vi "Format RunningInstancesItemType_LVXML_Loop.vi"(8 "error in (no error)":errorcluster, 10 "Siblings in":T2(array[cluster]), 11 "AWS_EC2 in":refnum<class "AWS_EC2.lvclass">) -> (0 "error out":errorcluster, 2 "Array":T3[](array[typedef]), 3 "AWS_EC2 out":refnum<class "AWS_EC2.lvclass">)   [LabVIEW 2014, in "AWS_EC2.lvlib" / "AWS_EC2.lvclass"]
uses:
  AWS_EC2.lvclass
  EC2 Datatypes/RunningInstancesItemsType.ctl
  EC2 Datatypes/InstanceStateType.ctl
  EC2 Datatypes/ProductCodeSetItemType.ctl
  EC2 Datatypes/PlacementResponseType.ctl
  EC2 Datatypes/GroupItemTypeSet.ctl
  EC2 Datatypes/GroupItemType.ctl
  EC2 Datatypes/StateReasonType.ctl
  EC2 Datatypes/InstanceBlockDeviceMappingResponseItemType.ctl
  EC2 Datatypes/EbsInstanceBlockDeviceMappingResponseType.ctl
  EC2 Datatypes/ResourceTagSetItemType.ctl
  EC2 Datatypes/InstanceNetworkInterfaceSetItemType.ctl
  EC2 Datatypes/InstanceNetworkInterfaceAttachmentType.ctl
  EC2 Datatypes/InstanceNetworkInterfaceAssociationType.ctl
  EC2 Datatypes/InstancePrivateIpAddressesSetItemType.ctl
  EC2 Datatypes/IamInstanceProfileResponseType.ctl
  lv-xml-parser/r0/trunk/VI Source/EventType.ctl
  AWS_EC2.lvlib
  AWS Core Lib/VI Source/AWS_Core.lvlib
  lv-xml-parser/r0/trunk/VI Source/LV XML Parser.lvlib
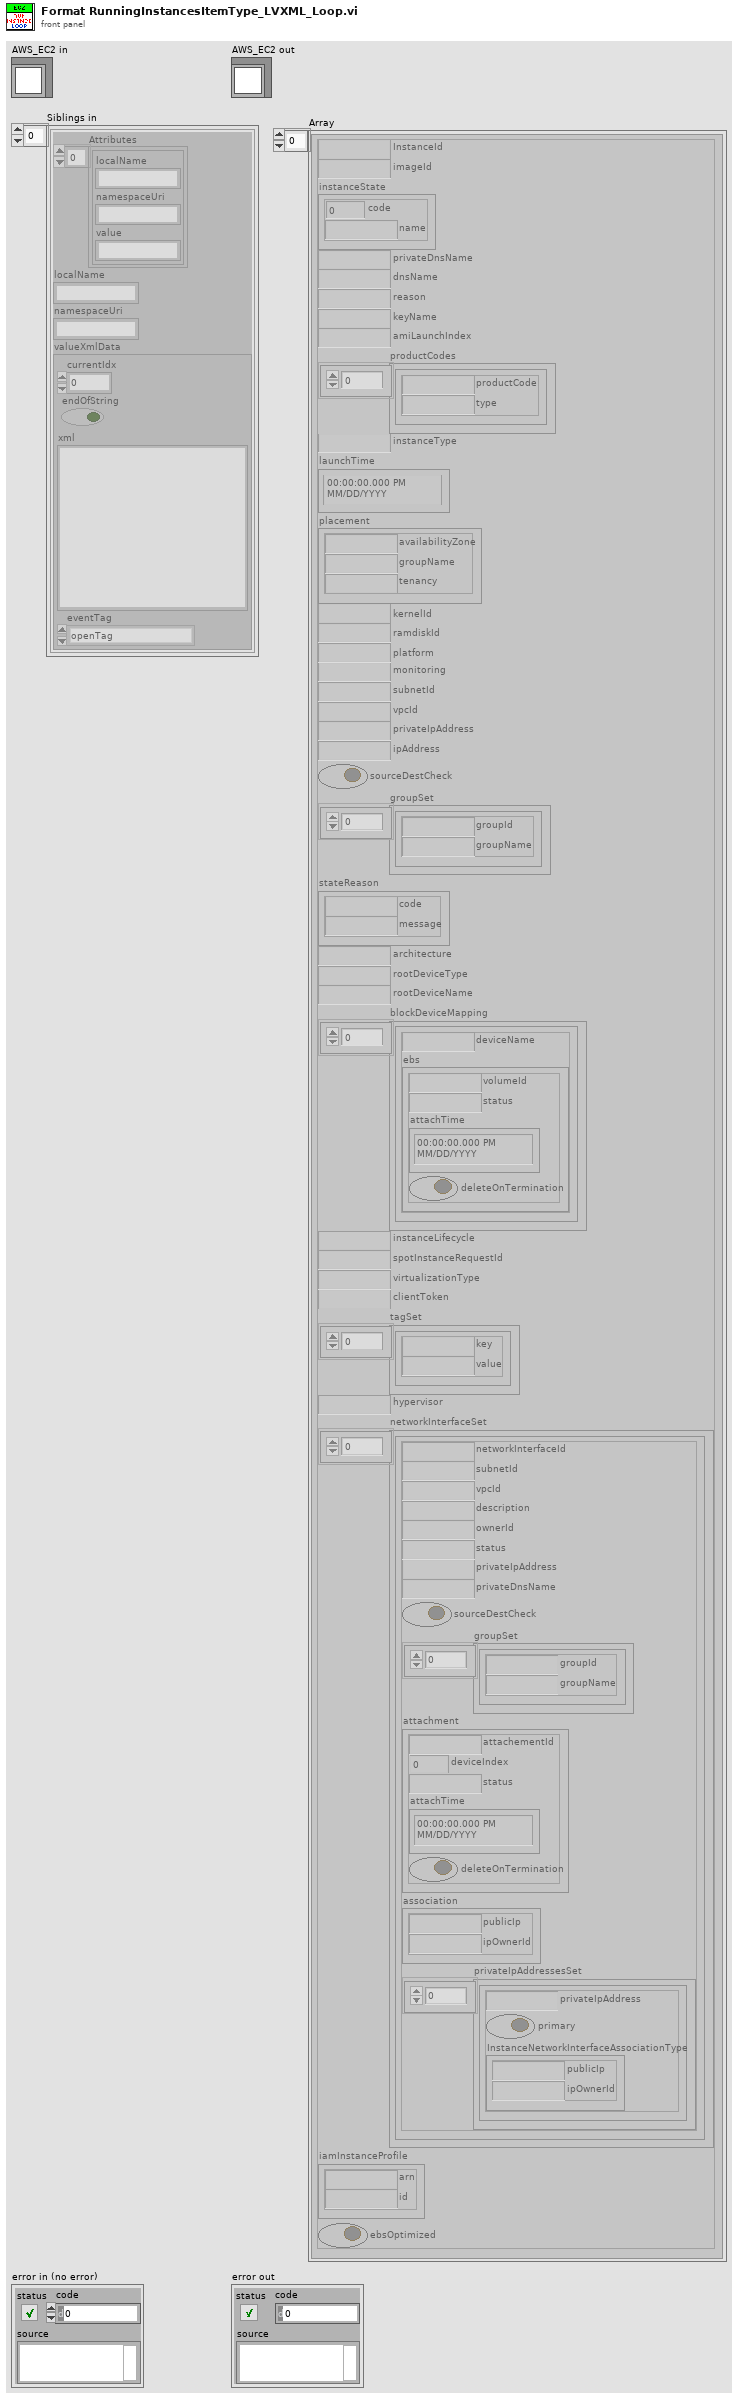
[diagram p1: front panel]
types:
  T1 = typedef "LV XML Parser.lvlib/EventType.ctl" = enum16{"openTag", "endOpenTag", "closeTag", "comment", "endComment", "endOfFile", "attribute", "startXml", "selfClosingTag"}
  T2 = cluster{"Attributes":cluster{"localName":string, "namespaceUri":string, "value":string}[], "localName":string, "namespaceUri":string, "valueXmlData":cluster{"currentIdx":i32, "endOfString":bool, "xml":string, "eventTag":T1}}[]
  T3 = typedef "AWS_EC2.lvlib/RunningInstancesItemsType.ctl" = cluster{"InstanceId":string, "imageId":string, "instanceState":T4, "privateDnsName":string, "dnsName":string, "reason":string, "keyName":string, "amiLaunchIndex":string, "productCodes":T5[], "instanceType":string, "launchTime":timestamp, "placement":T6, "kernelId":string, "ramdiskId":string, "platform":string, "monitoring":string, "subnetId":string, "vpcId":string, "privateIpAddress":string, "ipAddress":string, "sourceDestCheck":bool, "groupSet":T7, "stateReason":T9, "architecture":string, "rootDeviceType":string, "rootDeviceName":string, "blockDeviceMapping":T10[], "instanceLifecycle":string, "spotInstanceRequestId":string, "virtualizationType":string, "clientToken":string, "tagSet":T12[], "hypervisor":string, "networkInterfaceSet":T13[], "iamInstanceProfile":T17, "ebsOptimized":bool}
  T4 = typedef "AWS_EC2.lvlib/InstanceStateType.ctl" = cluster{"code":i16, "name":string}
  T5 = typedef "AWS_EC2.lvlib/ProductCodeSetItemType.ctl" = cluster{"productCode":string, "type":string}
  T6 = typedef "AWS_EC2.lvlib/PlacementResponseType.ctl" = cluster{"availabilityZone":string, "groupName":string, "tenancy":string}
  T7 = typedef "AWS_EC2.lvlib/GroupItemTypeSet.ctl" = T8[]
  T8 = typedef "AWS_EC2.lvlib/GroupItemType.ctl" = cluster{"groupId":string, "groupName":string}
  T9 = typedef "AWS_EC2.lvlib/StateReasonType.ctl" = cluster{"code":string, "message":string}
  T10 = typedef "AWS_EC2.lvlib/InstanceBlockDeviceMappingResponseItemType.ctl" = cluster{"deviceName":string, "ebs":T11}
  T11 = typedef "AWS_EC2.lvlib/EbsInstanceBlockDeviceMappingResponseType.ctl" = cluster{"volumeId":string, "status":string, "attachTime":timestamp, "deleteOnTermination":bool}
  T12 = typedef "AWS_EC2.lvlib/ResourceTagSetItemType.ctl" = cluster{"key":string, "value":string}
  T13 = typedef "AWS_EC2.lvlib/InstanceNetworkInterfaceSetItemType.ctl" = cluster{"networkInterfaceId":string, "subnetId":string, "vpcId":string, "description":string, "ownerId":string, "status":string, "privateIpAddress":string, "privateDnsName":string, "sourceDestCheck":bool, "groupSet":T7, "attachment":T14, "association":T15, "privateIpAddressesSet":T16[]}
  T14 = typedef "AWS_EC2.lvlib/InstanceNetworkInterfaceAttachmentType.ctl" = cluster{"attachementId":string, "deviceIndex":i32, "status":string, "attachTime":timestamp, "deleteOnTermination":bool}
  T15 = typedef "AWS_EC2.lvlib/InstanceNetworkInterfaceAssociationType.ctl" = cluster{"publicIp":string, "ipOwnerId":string}
  T16 = typedef "AWS_EC2.lvlib/InstancePrivateIpAddressesSetItemType.ctl" = cluster{"privateIpAddress":string, "primary":bool, "InstanceNetworkInterfaceAssociationType":T15}
  T17 = typedef "AWS_EC2.lvlib/IamInstanceProfileResponseType.ctl" = cluster{"arn":string, "id":string}
  T18 = cluster{"Attributes":cluster{"localName":string, "namespaceUri":string, "value":string}[], "localName":string, "namespaceUri":string, "valueXmlData":cluster{"currentIdx":i32, "endOfString":bool, "xml":string, "eventTag":T1}}
  T19 = cluster{"currentIdx":i32, "endOfString":bool, "xml":string, "eventTag":T1}
  T20 = cluster{"namespaceUri":string, "localName":string}
  T21 = cluster{"Attributes":cluster{"localName":string, "namespaceUri":string, "value":string}[], "localName":string, "namespaceUri":string, "valueXmlData":cluster{"currentIdx":i64, "endOfString":bool, "xml":string, "eventTag":T1}}[]
  T22 = cluster{"currentIdx":i64, "endOfString":bool, "xml":string, "eventTag":T1}
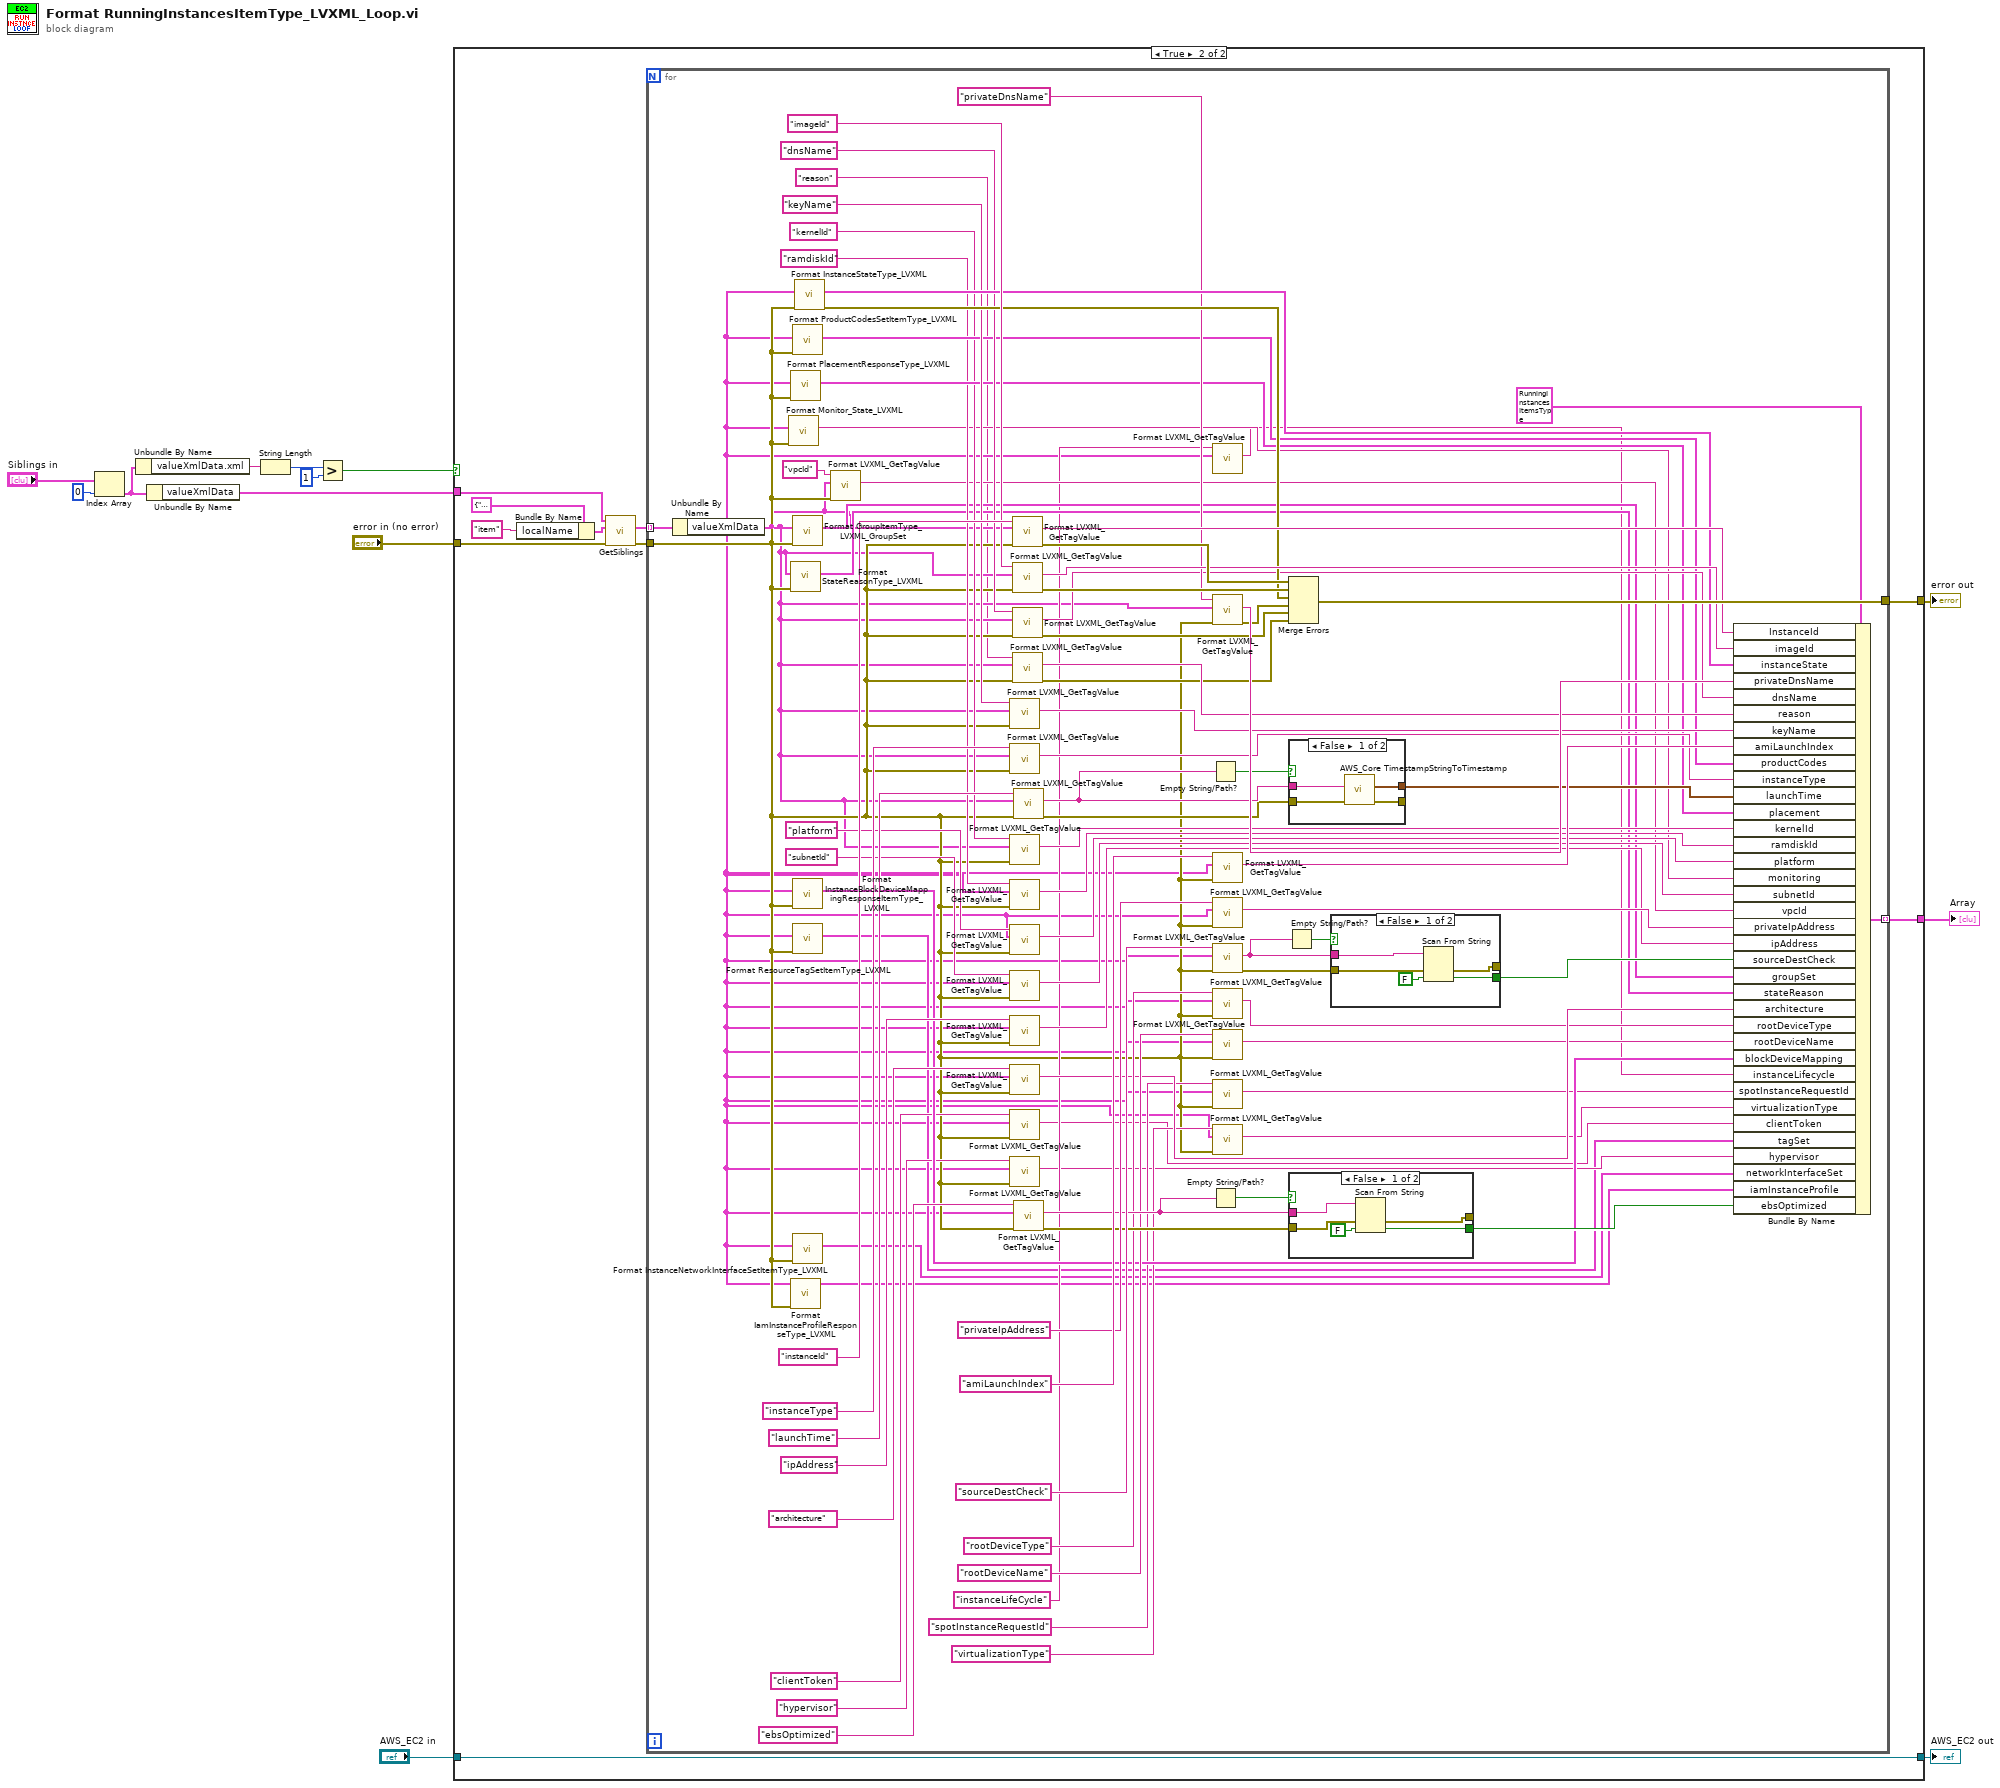
[diagram p0: block diagram]
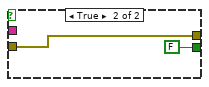
[diagram p3: hidden frame]
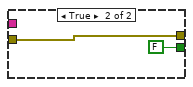
[diagram p4: hidden frame]
diagram:
  n1 = Index Array(array="Siblings in", index=0) -> (element=w10:T18)
  n2 = Unbundle By Name(w10) -> ("valueXmlData.xml"=w9:string)
  n3 = Unbundle By Name(w10) -> ("valueXmlData"=w8:T19)
  n4 = String Length(string=w9) -> (length=w5:i32)
  n5 = Greater?(x=w5, y=1) -> (0:w7:bool)
  n6 = case shown="True" w7 {
    tunnel: [w15 w24] -> w1
    tunnel: "error in (no error)" -> [w15 w19]
    tunnel: w8 -> [_ w18]
    tunnel: "AWS_EC2 in" -> [w14 w17]
    tunnel: [w14 w17] -> w12
    tunnel: [_ w16] -> w13
    frame False {
    }
    frame True {
      n7 = Bundle By Name(cluster=T20 {"namespaceUri"="", "localName"=""} ("limitToTag"), "localName"="item" ("Tag name")) -> (w21:T20)
      n8 = call "GetSiblings.vi"("error in (no error)"=w19, "limitToTag"=w21, "xmlData"=w18) -> ("error out"=w25:errorcluster, "Siblings"=w22:T21)  [unwired: 7 in]
      n9 = for {
        tunnel: w22 -> [w108] mode=indexing
        tunnel: [w107] -> w24
        tunnel: w25 -> [w29]
        tunnel: [w99] -> w16 mode=indexing
        n10 = Unbundle By Name(w108) -> ("valueXmlData"=w28:T22)
        n11 = call "Format Monitor_State_LVXML.vi"("xmlData in"=w28, "error in (no error)"=w29) -> ("Value"=w69:string)  [unwired: 7 in, 1 out]
        n12 = call "Format PlacementResponseType_LVXML.vi"("error in (no error)"=w29, "valueXmlData in"=w28) -> ("PlacementResponseType"=w76:T6)  [unwired: 7 in, 2 out]
        n13 = call "Format StateReasonType_LVXML.vi"("error in (no error)"=w29, "xmlData in"=w28) -> ("StateReasonType"=w49:T9)  [unwired: 7 in, 2 out]
        n14 = call "Format IamInstanceProfileResponseType_LVXML.vi"("error in (no error)"=w29, "xmlData in"=w28) -> ("IamInstanceProfileResponseType"=w27:T17)  [unwired: 8 in, 1 out]
        n15 = call "Format ProductCodesSetItemType_LVXML.vi"("error in (no error)"=w29, "valueXmlData in"=w28) -> ("Array"=w84:T5[])  [unwired: 7 in, 2 out]
        n16 = call "Format GroupItemType_LVXML_GroupSet.vi"("error in (no error)"=w29, "valueXmlData"=w28) -> ("Array"=w50:T8[])  [unwired: 7 in, 2 out]
        n17 = call "Format InstanceBlockDeviceMappingResponseItemType_LVXML.vi"("error in (no error)"=w29, "valueXmlData in"=w28) -> ("Array"=w42:T10[])  [unwired: 7 in, 2 out]
        n18 = call "Format ResourceTagSetItemType_LVXML.vi"("error in (no error)"=w29, "valueXmlData in"=w28) -> ("Array"=w31:T12[])  [unwired: 7 in, 2 out]
        n19 = call "Format InstanceNetworkInterfaceSetItemType_LVXML.vi"("error in (no error)"=w29, "valueXmlData in"=w28) -> ("Array"=w30:T13[])  [unwired: 7 in, 2 out]
        n20 = call "Format InstanceStateType_LVXML.vi"("error in (no error)"=w29, "xmlData"=w28) -> ("error out"=w97:errorcluster, "InstanceStateType"=w98:T4)  [unwired: 7 in, 1 out]
        n21 = call "Format LVXML_GetTagValue.vi"("error in (no error)"=w29, "xmlDataIn"=w28, "Tag name"="vpcId") -> ("Value"=w65:string)  [unwired: 6 in, 2 out]
        n22 = call "Format LVXML_GetTagValue.vi"("error in (no error)"=w29, "xmlDataIn"=w28, "Tag name"="keyName") -> ("Value"=w87:string)  [unwired: 6 in, 2 out]
        n23 = call "Format LVXML_GetTagValue.vi"("error in (no error)"=w29, "xmlDataIn"=w28, "Tag name"="instanceType") -> ("Value"=w82:string)  [unwired: 6 in, 2 out]
        n24 = call "Format LVXML_GetTagValue.vi"("error in (no error)"=w29, "xmlDataIn"=w28, "Tag name"="kernelId") -> ("Value"=w73:string)  [unwired: 6 in, 2 out]
        n25 = call "Format LVXML_GetTagValue.vi"("error in (no error)"=w29, "xmlDataIn"=w28, "Tag name"="ramdiskId") -> ("Value"=w71:string)  [unwired: 6 in, 2 out]
        n26 = call "Format LVXML_GetTagValue.vi"("error in (no error)"=w29, "xmlDataIn"=w28, "Tag name"="platform") -> ("Value"=w70:string)  [unwired: 6 in, 2 out]
        n27 = call "Format LVXML_GetTagValue.vi"("error in (no error)"=w29, "xmlDataIn"=w28, "Tag name"="subnetId") -> ("Value"=w67:string)  [unwired: 6 in, 2 out]
        n28 = call "Format LVXML_GetTagValue.vi"("error in (no error)"=w29, "xmlDataIn"=w28, "Tag name"="ipAddress") -> ("Value"=w61:string)  [unwired: 6 in, 2 out]
        n29 = call "Format LVXML_GetTagValue.vi"("error in (no error)"=w29, "xmlDataIn"=w28, "Tag name"="architecture") -> ("Value"=w45:string)  [unwired: 6 in, 2 out]
        n30 = call "Format LVXML_GetTagValue.vi"("error in (no error)"=w29, "xmlDataIn"=w28, "Tag name"="clientToken") -> ("Value"=w34:string)  [unwired: 6 in, 2 out]
        n31 = call "Format LVXML_GetTagValue.vi"("error in (no error)"=w29, "xmlDataIn"=w28, "Tag name"="hypervisor") -> ("Value"=w32:string)  [unwired: 6 in, 2 out]
        n32 = call "Format LVXML_GetTagValue.vi"("error in (no error)"=w29, "xmlDataIn"=w28, "Tag name"="instanceId") -> ("error out"=w104:errorcluster, "Value"=w101:string)  [unwired: 6 in, 1 out]
        n33 = call "Format LVXML_GetTagValue.vi"("error in (no error)"=w29, "xmlDataIn"=w28, "Tag name"="imageId") -> ("error out"=w103:errorcluster, "Value"=w100:string)  [unwired: 6 in, 1 out]
        n34 = call "Format LVXML_GetTagValue.vi"("error in (no error)"=w29, "xmlDataIn"=w28, "Tag name"="dnsName") -> ("error out"=w90:errorcluster, "Value"=w93:string)  [unwired: 6 in, 1 out]
        n35 = call "Format LVXML_GetTagValue.vi"("error in (no error)"=w29, "xmlDataIn"=w28, "Tag name"="reason") -> ("error out"=w89:errorcluster, "Value"=w92:string)  [unwired: 6 in, 1 out]
        n36 = call "Format LVXML_GetTagValue.vi"("error in (no error)"=w29, "xmlDataIn"=w28, "Tag name"="launchTime") -> ("error out"=w77:errorcluster, "Value"=w80:string)  [unwired: 6 in, 1 out]
        n37 = call "Format LVXML_GetTagValue.vi"("error in (no error)"=w29, "xmlDataIn"=w28, "Tag name"="ebsOptimized") -> ("error out"=w55:errorcluster, "Value"=w54:string)  [unwired: 6 in, 1 out]
        n38 = Empty String/Path?(string/path=w80) -> (empty?=w81:bool)
        n39 = Empty String/Path?(string/path=w54) -> (empty?=w53:bool)
        n40 = call "Format LVXML_GetTagValue.vi"("xmlDataIn"=w28, "Tag name"="instanceLifeCycle") -> ("Value"=w37:string)  [unwired: 7 in, 2 out]
        n41 = call "Format LVXML_GetTagValue.vi"("error in (no error)"=w29, "xmlDataIn"=w28, "Tag name"="privateDnsName") -> ("error out"=w91:errorcluster, "Value"=w95:string)  [unwired: 6 in, 1 out]
        n42 = call "Format LVXML_GetTagValue.vi"("error in (no error)"=w29, "xmlDataIn"=w28, "Tag name"="amiLaunchIndex") -> ("Value"=w85:string)  [unwired: 6 in, 2 out]
        n43 = call "Format LVXML_GetTagValue.vi"("error in (no error)"=w29, "xmlDataIn"=w28, "Tag name"="privateIpAddress") -> ("Value"=w63:string)  [unwired: 6 in, 2 out]
        n44 = call "Format LVXML_GetTagValue.vi"("error in (no error)"=w29, "xmlDataIn"=w28, "Tag name"="sourceDestCheck") -> ("error out"=w57:errorcluster, "Value"=w58:string)  [unwired: 6 in, 1 out]
        n45 = call "Format LVXML_GetTagValue.vi"("error in (no error)"=w29, "xmlDataIn"=w28, "Tag name"="rootDeviceType") -> ("Value"=w44:string)  [unwired: 6 in, 2 out]
        n46 = call "Format LVXML_GetTagValue.vi"("error in (no error)"=w29, "xmlDataIn"=w28, "Tag name"="rootDeviceName") -> ("Value"=w43:string)  [unwired: 6 in, 2 out]
        n47 = call "Format LVXML_GetTagValue.vi"("error in (no error)"=w29, "xmlDataIn"=w28, "Tag name"="spotInstanceRequestId") -> ("Value"=w36:string)  [unwired: 6 in, 2 out]
        n48 = call "Format LVXML_GetTagValue.vi"("error in (no error)"=w29, "xmlDataIn"=w28, "Tag name"="virtualizationType") -> ("Value"=w35:string)  [unwired: 6 in, 2 out]
        n49 = Empty String/Path?(string/path=w58) -> (empty?=w59:bool)
        n50 = Merge Errors(w104, w103, w97, w91, w90, w89) -> (w107:errorcluster)
        n51 = case shown="False" w81 {
          tunnel: w80 -> [w126 _]
          tunnel: [w125 _] -> w78
          tunnel: w77 -> [w124 w127]
          tunnel: [w123 w127] -> _
          frame False {
            n52 = call "AWS_Core TimestampStringToTimestamp.vi"("error in"=w124, "AWS Timestamp String"=w126) -> ("error out"=w123:errorcluster, "Time Stamp Control"=w125:timestamp)  [unwired: 8 in]
          }
          frame True {
          }
        }
        n53 = case shown="False" w53 {
          tunnel: [w113 w115] -> _
          tunnel: [w112 FALSE] -> w51
          tunnel: w55 -> [w110 w115]
          tunnel: w54 -> [w109 _]
          frame False {
            n54 = Scan From String(input string=w109, error in=w110, default 1=FALSE) -> (error out=w113:errorcluster, output 1=w112:bool)  [unwired: 2 in, 2 out]
          }
          frame True {
          }
        }
        n55 = case shown="False" w59 {
          tunnel: [w120 w122] -> _
          tunnel: [w119 FALSE] -> w56
          tunnel: w57 -> [w117 w122]
          tunnel: w58 -> [w116 _]
          frame False {
            n56 = Scan From String(input string=w116, error in=w117, default 1=FALSE) -> (error out=w120:errorcluster, output 1=w119:bool)  [unwired: 2 in, 2 out]
          }
          frame True {
          }
        }
        n57 = Bundle By Name(cluster=T3 {"InstanceId"="", "imageId"="", "instanceState"={"code"=0, "name"=""}, "privateDnsName"="", "dnsName"="", "reason"="", "keyName"="", "amiLaunchIndex"="", "productCodes"=[], "instanceType"="", "launchTime"=timestamp(0 s since 1904-01-01), "placement"={"availabilityZone"="", "groupName"="", "tenancy"=""}, "kernelId"="", "ramdiskId"="", "platform"="", "monitoring"="", "subnetId"="", "vpcId"="", "privateIpAddress"="", "ipAddress"="", "sourceDestCheck"=FALSE, "groupSet"=[], "stateReason"={"code"="", "message"=""}, "architecture"="", "rootDeviceType"="", "rootDeviceName"="", "blockDeviceMapping"=[], "instanceLifecycle"="", "spotInstanceRequestId"="", "virtualizationType"="", "clientToken"="", "tagSet"=[], "hypervisor"="", "networkInterfaceSet"=[], "iamInstanceProfile"={"arn"="", "id"=""}, "ebsOptimized"=FALSE} ("RunningInstancesItemType"), "InstanceId"=w101, "imageId"=w100, "instanceState"=w98, "privateDnsName"=w95, "dnsName"=w93, "reason"=w92, "keyName"=w87, "amiLaunchIndex"=w85, "productCodes"=w84, "instanceType"=w82, "launchTime"=w78, "placement"=w76, "kernelId"=w73, "ramdiskId"=w71, "platform"=w70, "monitoring"=w69, "subnetId"=w67, "vpcId"=w65, "privateIpAddress"=w63, "ipAddress"=w61, "sourceDestCheck"=w56, "groupSet"=w50, "stateReason"=w49, "architecture"=w45, "rootDeviceType"=w44, "rootDeviceName"=w43, "blockDeviceMapping"=w42, "instanceLifecycle"=w37, "spotInstanceRequestId"=w36, "virtualizationType"=w35, "clientToken"=w34, "tagSet"=w31, "hypervisor"=w32, "networkInterfaceSet"=w30, "iamInstanceProfile"=w27, "ebsOptimized"=w51) -> (w99:T3)
      }
    }
  }
  "Array" <- w13
  "AWS_EC2 out" <- w12
  "error out" <- w1
